vi "New Schedule Reset.vi"(8 "error in (no error)":errorcluster, 9 "DAQ Control":T1, 10 "Schedule":refnum<class "Schedule.lvclass">, 11 "Monkey in":refnum<class "Monkey.lvclass">) -> (0 "error out":errorcluster, 3 "Monkey out":refnum<class "Monkey.lvclass">)   [LabVIEW 2020, in "Monkey.lvlib" / "Monkey.lvclass"]
doc: "Reset all the flags at the beginning of the schedule"
uses:
  Monkey.lvclass
  Run Utilities/Schedule/Schedule.lvclass
  Run Utilities/TypeDefs/DAQ Control.ctl
  Run Utilities/TypeDefs/Script Checker Result.ctl
  Monkey.lvclass/Monkey.ctl
  Run Utilities/Run Block/Run Block.lvclass
  Run Utilities/Run Utilities.lvlib
  TALOS/TALOS_PPL.lvlibp
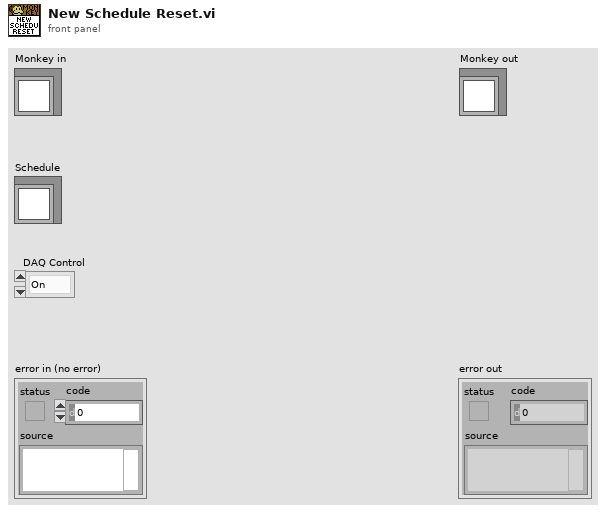
[diagram p1: front panel]
types:
  T1 = typedef "Run Utilities.lvlib/DAQ Control.ctl" = enum16{"On", "Off", "External"}
  T2 = typedef "Run Utilities.lvlib/Script Checker Result.ctl" = enum16{"Passed", "Failed", "Empty"}
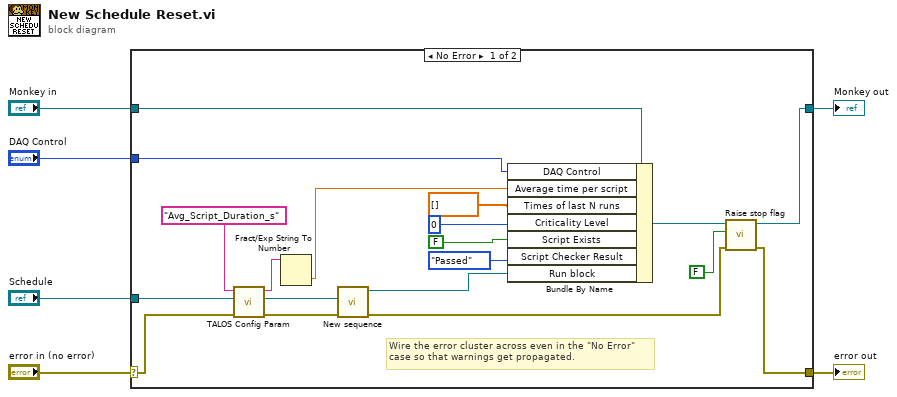
[diagram p0: block diagram]
diagram:
  n1 = case shown="No Error" "error in (no error)" {
    selector: "error in (no error)" -> [w10 w26]
    tunnel: [w14 w26] -> w5
    tunnel: [w12 w25] -> w3
    tunnel: "Monkey in" -> [w24 w25]
    tunnel: "Schedule" -> [w23 _]
    tunnel: "DAQ Control" -> [w21 _]
    frame No Error {
      # "Wire the error cluster across even in the \"No Error\"\ncase so that warnings get propagated."
      n2 = call "TALOS Config Param.vi"("error in (no error)"=w10, "Parameter Name"="Avg_Script_Duration_s") -> ("error out"=w11:errorcluster, "Output"=w8:string)  [unwired: 8 in]
      n3 = Fract/Exp String To Number(string=w8) -> (number=w7:dbl)  [unwired: 3 in, 1 out]
      n4 = call "New sequence.vi"("error in (no error)"=w11, "Schedule"=w23) -> ("error out"=w15:errorcluster, "Run Block out"=w22:refnum<class "Run Block.lvclass">)  [unwired: 8 in]
      n5 = Bundle By Name(cluster=w24, "DAQ Control"=w21, "Average time per script"=w7, "Times of last N runs"=dbl[] [], "Criticality Level"=u8 0, "Script Exists"=FALSE, "Script Checker Result"=Script_Checker_Result."Passed", "Run block"=w22) -> (w13:refnum<class "Monkey.lvclass">)
      n6 = call-dynamic "Raise stop flag.vi"("error in (no error)"=w15, "on/off"=FALSE, "Monkey in"=w13) -> ("error out"=w14:errorcluster, "Monkey out"=w12:refnum<class "Monkey.lvclass">)  [unwired: 7 in]
    }
    frame Error {
    }
  }
  "error out" <- w5
  "Monkey out" <- w3
